vi "Write UI Ref Total Counts.vi"(8 "error in (no error)":errorcluster, 10 "UI Ref Total Counts":refnum<vi>, 11 "Analyze Results Total Counts in":refnum<class "Analyze Results Total Counts.lvclass">) -> (0 "error out":errorcluster, 3 "Analyze Results Total Counts out":refnum<class "Analyze Results Total Counts.lvclass">)   [LabVIEW 2014, in "Analyze Results Total Counts.lvclass"]
uses:
  Analyze Results Total Counts.lvclass
  Analyze Results Total Counts.lvclass/Analyze Results Total Counts.ctl
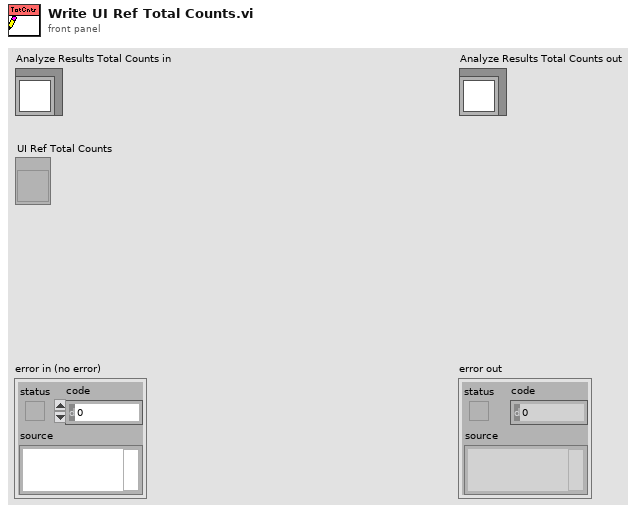
[diagram p1: front panel]
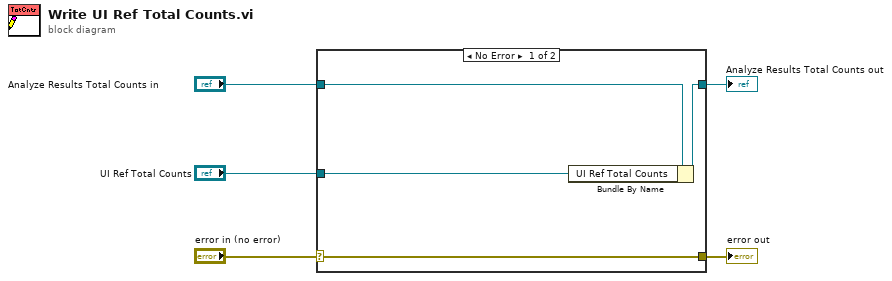
[diagram p0: block diagram]
diagram:
  n1 = case shown="No Error" "error in (no error)" {
    selector: "error in (no error)" -> [w9 w10]
    tunnel: [w9 w10] -> w4
    tunnel: [w7 w11] -> w2
    tunnel: "Analyze Results Total Counts in" -> [w8 w11]
    tunnel: "UI Ref Total Counts" -> [w6 _]
    frame No Error {
      n2 = Bundle By Name(cluster=w8, "UI Ref Total Counts"=w6) -> (w7:refnum<class "Analyze Results Total Counts.lvclass">)
    }
    frame Error {
    }
  }
  "error out" <- w4
  "Analyze Results Total Counts out" <- w2
